vi "Accelerometer.vi"   [LabVIEW 2016]
uses:
  <vilib>/rvi/eio/common/nirviEmuTemplateMethod_errors.vi
  <vilib>/eio/EIONode/EIONode.xnode
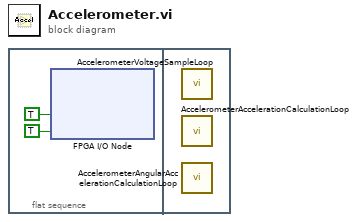
[diagram p0: block diagram]
diagram:
  n1 = flat-sequence {
    frame #0 {
      n2 = xnode "FPGA I/O Node"("Mod1/Start"=TRUE, "Mod2/Start"=TRUE) -> ()  [unwired: 3 in, 4 out]
    }
    frame #1 {
      n3 = call "AccelerometerVoltageSampleLoop.vi"() -> ()  [unwired: 12 in]
      n4 = call "AccelerometerAccelerationCalculationLoop.vi"() -> ()  [unwired: 12 in]
      n5 = call "AccelerometerAngularAccelerationCalculationLoop.vi"() -> ()  [unwired: 12 in]
    }
  }
